vi "Launcher.vi"   [LabVIEW 2024, in "Application.lvlib"]
uses:
  Application.lvlib
  GUI/GUI.lvlib
types:
  T1 = enum32{"Invalid", "Standard", "Closed", "Hidden", "Minimized", "Maximized"}
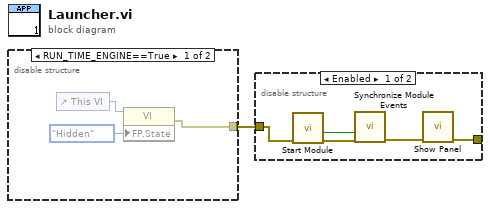
[diagram p0: block diagram]
diagram:
  n1 = disable-structure shown="RUN_TIME_ENGINE==True" {
    disable-tunnel: [w2 _] -> w1
    frame condition #0 {
      n2 = control-ref of="This VI"() -> (w4:refnum<vi>)
      n3 = property class="VI"(reference=w4, "FP.State"=T1."Hidden" ("Front Panel Window:State")) -> (error out=w2:errorcluster)  [unwired: 1 in, 1 out]
    }
    frame condition #1 (active) {
    }
  }
  n4 = disable-structure shown="Enabled" {
    disable-tunnel: [w6 _] -> _
    disable-tunnel: w1 -> [w5 _]
    frame Enabled {
      n5 = call "Start Module.vi"("error in"=w5) -> ("error out"=w8:errorcluster, "Wait for Event Sync?"=w9:bool)  [unwired: 6 in, 3 out]
      n6 = call "Synchronize Module Events.vi"("error in"=w8, "Wait for Event Sync?"=w9) -> ("error out"=w7:errorcluster)  [unwired: 9 in]
      n7 = call "Show Panel.vi"("error in"=w7) -> ("error out"=w6:errorcluster)  [unwired: 10 in]
    }
    frame Disabled {
    }
  }
